vi "writetangentsettings.vi"(3 "Path":path, 4 "?":T1, 5 "error in (no error)":errorcluster) -> (0 "error out":errorcluster, 1 "Path 2":path)   [LabVIEW 2012]
uses:
  <vilib>/Utility/config.llb/Write Key (Double).vi
  <vilib>/Utility/config.llb/NI_LVConfig.lvlib
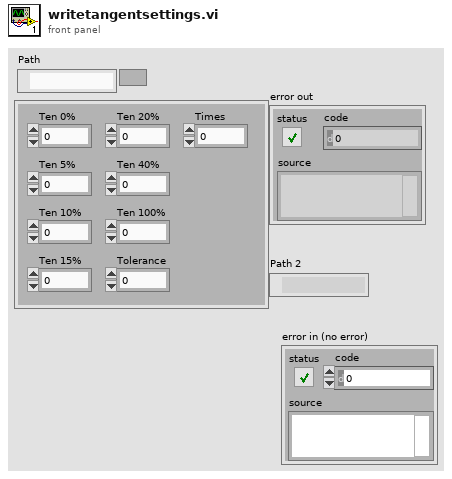
[diagram p1: front panel]
types:
  T1 = cluster{"Ten 0%":dbl, "Ten 5%":dbl, "Ten 10%":dbl, "Ten 15%":dbl, "Tolerance":dbl, "Ten 20%":dbl, "Ten 40%":dbl, "Ten 100%":dbl, "Times":dbl}
  T2 = typedef "NI_LVConfig.lvlib/Config Data RefNum.ctl" = refnum<k1>
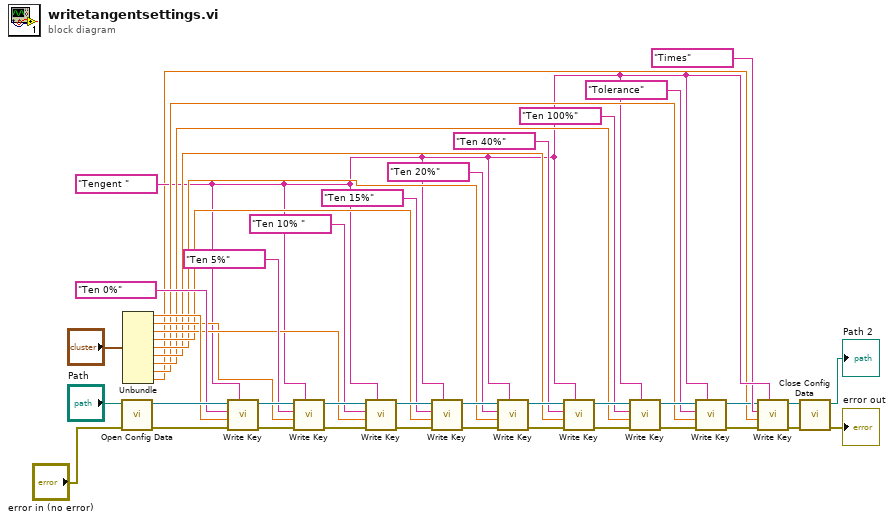
[diagram p0: block diagram]
diagram:
  w8 = "Tengent "
  n1 = call <vilib>:"Open Config Data.vi"("error in (no error)"="error in (no error)", "configuration file path"="Path") -> ("error out"=w37:errorcluster, "refnum"=w43:T2)  [unwired: 7 in, 1 out]
  n2 = Unbundle("?") -> ("Ten 0%"=w17:dbl, "Ten 5%"=w14:dbl, "Ten 10%"=w15:dbl, "Ten 15%"=w13:dbl, "Tolerance"=w12:dbl, "Ten 20%"=w11:dbl, "Ten 40%"=w10:dbl, "Ten 100%"=w9:dbl, "Times"=w2:dbl)
  n3 = call-poly <vilib>:"Write Key.vi"("section"=w8, "error in (no error)"=w37, "value"=w17, "key"="Ten 0%", "refnum"=w43) -> ("error out"=w16:errorcluster, "refnum out"=w42:T2)  [unwired: 4 in, 1 out]
  n4 = call-poly <vilib>:"Write Key.vi"("section"=w8, "error in (no error)"=w16, "value"=w14, "key"="Ten 5%", "refnum"=w42) -> ("error out"=w36:errorcluster, "refnum out"=w41:T2)  [unwired: 4 in, 1 out]
  n5 = call-poly <vilib>:"Write Key.vi"("section"=w8, "error in (no error)"=w36, "value"=w15, "key"="Ten 10% ", "refnum"=w41) -> ("error out"=w35:errorcluster, "refnum out"=w40:T2)  [unwired: 4 in, 1 out]
  n6 = call-poly <vilib>:"Write Key.vi"("section"=w8, "error in (no error)"=w35, "value"=w13, "key"="Ten 15%", "refnum"=w40) -> ("error out"=w34:errorcluster, "refnum out"=w39:T2)  [unwired: 4 in, 1 out]
  n7 = call-poly <vilib>:"Write Key.vi"("section"=w8, "error in (no error)"=w34, "value"=w12, "key"="Ten 20%", "refnum"=w39) -> ("error out"=w33:errorcluster, "refnum out"=w38:T2)  [unwired: 4 in, 1 out]
  n8 = call-poly <vilib>:"Write Key.vi"("section"=w8, "error in (no error)"=w33, "value"=w11, "key"="Ten 40%", "refnum"=w38) -> ("error out"=w22:errorcluster, "refnum out"=w24:T2)  [unwired: 4 in, 1 out]
  n9 = call-poly <vilib>:"Write Key.vi"("section"=w8, "error in (no error)"=w22, "value"=w10, "key"="Ten 100%", "refnum"=w24) -> ("error out"=w21:errorcluster, "refnum out"=w23:T2)  [unwired: 4 in, 1 out]
  n10 = call-poly <vilib>:"Write Key.vi"("section"=w8, "error in (no error)"=w21, "value"=w9, "key"="Tolerance", "refnum"=w23) -> ("error out"=w5:errorcluster, "refnum out"=w6:T2)  [unwired: 4 in, 1 out]
  n11 = call-poly <vilib>:"Write Key.vi"("section"=w8, "error in (no error)"=w5, "value"=w2, "key"="Times", "refnum"=w6) -> ("error out"=w3:errorcluster, "refnum out"=w4:T2)  [unwired: 4 in, 1 out]
  n12 = call <vilib>:"Close Config Data.vi"("error in (no error)"=w3, "refnum"=w4) -> ("error out"=→"error out":errorcluster, "file path"=→"Path 2":path)  [unwired: 8 in]
